vi "callPLC.vi"(8 "Error In":errorcluster, 11 "plcUDE":T1) -> (0 "Error Out":errorcluster)   [LabVIEW 2018]
uses:
  Modbus Module/src/controls/modbusUDE.ctl
  Modbus Module/src/controls/modbusData.ctl
  controls/readRegisterModbusCluster.ctl
  controls/controllerData.ctl
  UI Module/src/controls/mainAppElementsCluster.ctl
  Barcode Printer Module/src/controls/printData.ctl
  Barcode Scanner Module/src/controls/scanData.ctl
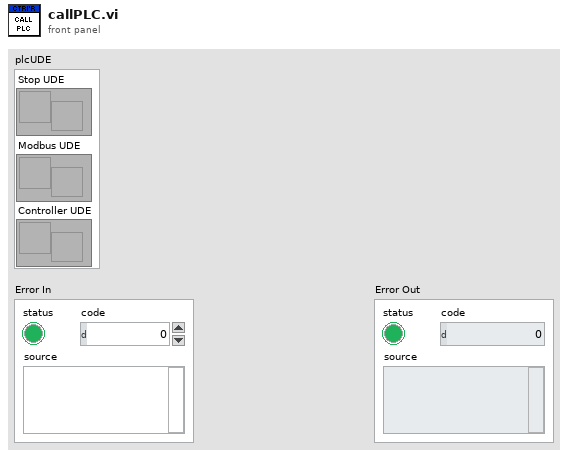
[diagram p1: front panel]
types:
  T1 = typedef "modbusUDE.ctl" = cluster{"Stop UDE":refnum<user-event>, "Modbus UDE":refnum<user-event>, "Controller UDE":refnum<user-event>}
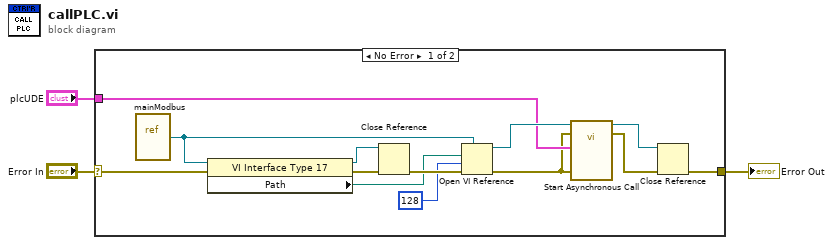
[diagram p0: block diagram]
diagram:
  n1 = case shown="No Error" "Error In" {
    selector: "Error In" -> [w16 w17]
    tunnel: [w7 w17] -> w2
    tunnel: "plcUDE" -> [w5 _]
    frame No Error {
      n2 = vi-ref "mainModbus.vi"() -> (w9:refnum<vi>)
      n3 = property class="VI Interface Type 17"(reference=w9, error in=w16) -> (reference out=w14:refnum<vi>, error out=w15:errorcluster, "Path"=w12:path)
      n4 = Close Reference(reference=w14, error in (no error)=w15) -> (error out=w13:errorcluster)
      n5 = Open VI Reference(type specifier VI Refnum (for type only)=w9, vi path=w12, options=128, error in (no error)=w13) -> (vi reference=w10:refnum<vi>, error out=w4:errorcluster)  [unwired: 2 in]
      n6 = call-by-ref "Start Asynchronous Call"(reference=w10, error in=w4, "Error In"=w4, "plcUDE"=w5) -> (reference out=w6:refnum<vi>, error out=w8:errorcluster)  [unwired: 9 in, 1 out]
      n7 = Close Reference(reference=w6, error in (no error)=w8) -> (error out=w7:errorcluster)
    }
    frame Error {
    }
  }
  "Error Out" <- w2
